vi "Memory.Pointer.Errors.Out of Bounds.vi"(7 "source vi name":string, 8 "error in (no error)":errorcluster, 9 "length":u64 format="%d bytes", 10 "offset":u64 format="%d bytes", 11 "pointer in":refnum<class "Memory.Pointer.lvclass">) -> (0 "error out":errorcluster, 3 "pointer out":refnum<class "Memory.Pointer.lvclass">)   [LabVIEW 2016, in "Memory Manager.lvlib" / "Memory.Pointer.lvclass"]
uses:
  Memory.Pointer.lvclass
  Typedefs/Memory.Pointer.Errors.ctl
  Memory.Pointer.lvclass/Memory.Pointer.ctl
  Submodules/Static Error Handling/Source/Library/VIs/Static Error Handling.Source Buffer.Write.Numeric.Scalar.Base10 (U64).vi
  Accessors/Get Size.vi
  Submodules/Static Error Handling/Source/Library/VIs/Static Error Handling.Error Cluster Constant.vi
  Submodules/Static Error Handling/Source/Library/VIs/Static Error Handling.Error Cluster Constant (256B).vi
  Submodules/Static Error Handling/Source/Library/VIs/Static Error Handling.Parameters.Status.Set.vi
  Submodules/Static Error Handling/Source/Library/VIs/Static Error Handling.Parameters.Code.Set.vi
  Submodules/Static Error Handling/Source/Library/VIs/Static Error Handling.Parameters.VI Source.Set.vi
  Constants/Memory.Constants.vi
  Constants/Memory.Constants.Library Name.vi
  Memory.Pointer.Errors.Get Info.vi
  Submodules/Static Error Handling/Source/Library/Static Error Handling.lvlib
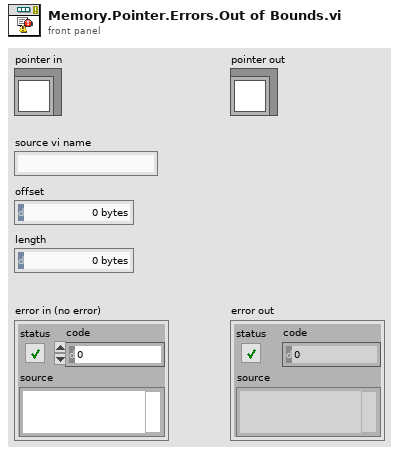
[diagram p1: front panel]
types:
  T1 = typedef "Memory Manager.lvlib/Memory.Pointer.lvclass/Memory.Pointer.Errors.ctl" = enum16{"Out of Bounds"}
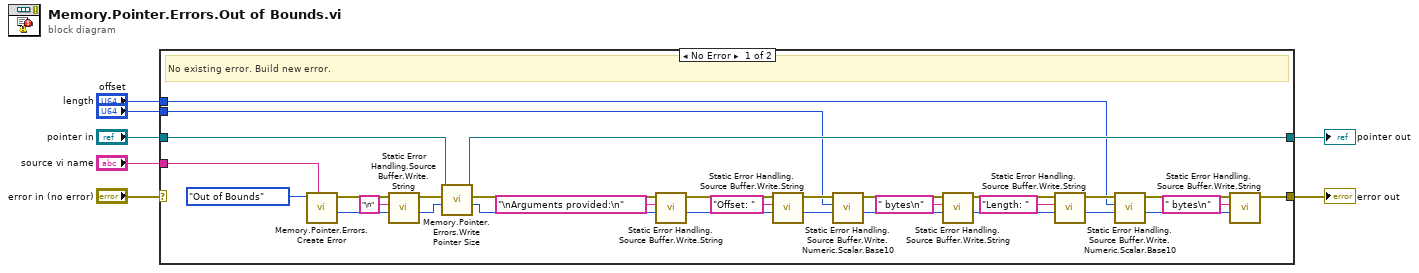
[diagram p0: block diagram]
diagram:
  n1 = case shown="No Error" "error in (no error)" {
    selector: "error in (no error)" -> [_ w40]
    tunnel: [w14 w40] -> w4
    tunnel: "offset" -> [w26 _]
    tunnel: "source vi name" -> [w30 _]
    tunnel: "pointer in" -> [w35 w39]
    tunnel: [w34 w39] -> w2
    tunnel: "length" -> [w13 _]
    frame No Error {
      # "No existing error. Build new error."
      n2 = call "Memory.Pointer.Errors.Create Error.vi"("source vi name"=w30, "error"=Memory.Pointer.Errors."Out of Bounds") -> ("new offset"=w32:i32, "error out"=w33:errorcluster)  [unwired: 8 in]
      n3 = call "Static Error Handling.Source Buffer.Write.String.vi"("offset"=w32, "string"="\n", "error in"=w33) -> ("new offset"=w36:i32, "error out"=w37:errorcluster)  [unwired: 7 in]
      n4 = call "Memory.Pointer.Errors.Write Pointer Size.vi"("offset"=w36, "error in"=w37, "pointer in"=w35) -> ("new offset"=w9:i32, "error out"=w12:errorcluster, "pointer out"=w34:refnum<class "Memory.Pointer.lvclass">)  [unwired: 6 in]
      n5 = call "Static Error Handling.Source Buffer.Write.String.vi"("offset"=w9, "string"="\nArguments provided:\n", "error in"=w12) -> ("new offset"=w10:i32, "error out"=w11:errorcluster)  [unwired: 7 in]
      n6 = call "Static Error Handling.Source Buffer.Write.String.vi"("offset"=w10, "string"="Offset: ", "error in"=w11) -> ("new offset"=w27:i32, "error out"=w28:errorcluster)  [unwired: 7 in]
      n7 = call-poly "Static Error Handling.Source Buffer.Write.Numeric.Scalar.Base10.vi"("offset"=w27, "value"=w26, "error in"=w28) -> ("new offset"=w23:i32, "error out"=w24:errorcluster)  [unwired: 7 in]
      n8 = call "Static Error Handling.Source Buffer.Write.String.vi"("offset"=w23, "string"=" bytes\n", "error in"=w24) -> ("new offset"=w15:i32, "error out"=w16:errorcluster)  [unwired: 7 in]
      n9 = call "Static Error Handling.Source Buffer.Write.String.vi"("offset"=w15, "string"="Length: ", "error in"=w16) -> ("new offset"=w20:i32, "error out"=w21:errorcluster)  [unwired: 7 in]
      n10 = call-poly "Static Error Handling.Source Buffer.Write.Numeric.Scalar.Base10.vi"("offset"=w20, "value"=w13, "error in"=w21) -> ("new offset"=w17:i32, "error out"=w18:errorcluster)  [unwired: 7 in]
      n11 = call "Static Error Handling.Source Buffer.Write.String.vi"("offset"=w17, "string"=" bytes\n", "error in"=w18) -> ("error out"=w14:errorcluster)  [unwired: 7 in, 1 out]
    }
    frame Error {
      # "Incoming error. Pass through."
    }
  }
  "error out" <- w4
  "pointer out" <- w2
